vi "Begin.vi"(8 "error in":errorcluster) -> (0 "error out":errorcluster)   [LabVIEW 2020]
doc: "Called before other user functions, this VI is expected to open initial I/O refnums, load in file data, and do all program initialization. Notice that the <B>error out</B> terminal is simply used for data flow. Wiring it to other structures or subVIs ensures that this VI runs first."
uses:
  <vilib>/Rock Robotics/WPI/DriverStation/WPI_DriverStationRobotMode2.ctl
  <vilib>/Rock Robotics/WPI/Joystick/WPI_JoystickDeviceEnum.ctl
  <vilib>/Rock Robotics/WPI/ThirdParty/REV Robotics/REVLib/Typedef/Spark MAX Motor Type.ctl
  <vilib>/Rock Robotics/WPI/SafetyOutput/WPI_SafetyOutputConfigMenu.ctl
  <vilib>/Rock Robotics/SystemInterfaces/DIO/FPGA_DIOChannel.ctl
  <vilib>/Rock Robotics/WPI/Encoder/WPI_EncoderType.ctl
  <vilib>/Rock Robotics/SystemInterfaces/spilib/spi_bus.ctl
  <vilib>/Rock Robotics/WPI/Solenoid/WPI_SolenoidChannel.ctl
  <vilib>/Rock Robotics/WPI/ThirdParty/REV Robotics/REVLib/Typedef/Spark MAX Idle Mode.ctl
  <vilib>/Rock Robotics/WPI/ThirdParty/Phoenix-LabVIEW/Motor Controller/Controls/CTRE_Phoenix_MotorControl_ControlMode.ctl
  <vilib>/Rock Robotics/WPI/DriverStation/WPI_DriverStationAllianceInfo.ctl
  <vilib>/Rock Robotics/SystemInterfaces/i2clib/i2c_bus.ctl
  Robot Global Data.vi
  <vilib>/Rock Robotics/Network Tables/NT Write String Array.vi
  <vilib>/Rock Robotics/WPI/Counter/WPI_CounterDigitalInputToDigitalSource.vi
  <vilib>/Rock Robotics/WPI/Gyro/WPI_GyroXRS450_SPI_Open.vi
  <vilib>/Rock Robotics/WPI/Solenoid/WPI_SolenoidOpenDouble.vi
  <vilib>/Rock Robotics/WPI/Switch/WPI_SwitchOpenLimit.vi
  Global Variable/StateMachineOperation.vi
  <vilib>/Rock Robotics/WPI/Utilities/WPI_GetSetVariantRefNum.vi
panel:
  in  "Nothing":cluster{"R":dbl, "G":dbl, "B":dbl}={"R"=0.197, "G"=0.561, "B"=0.24}
  in  "Red Calibration":cluster{"R":dbl, "G":dbl, "B":dbl}={"R"=0.561, "G"=0.323, "B"=0.114}
  in  "Blue Calibration":cluster{"R":dbl, "G":dbl, "B":dbl}={"R"=0.143, "G"=0.427, "B"=0.429}
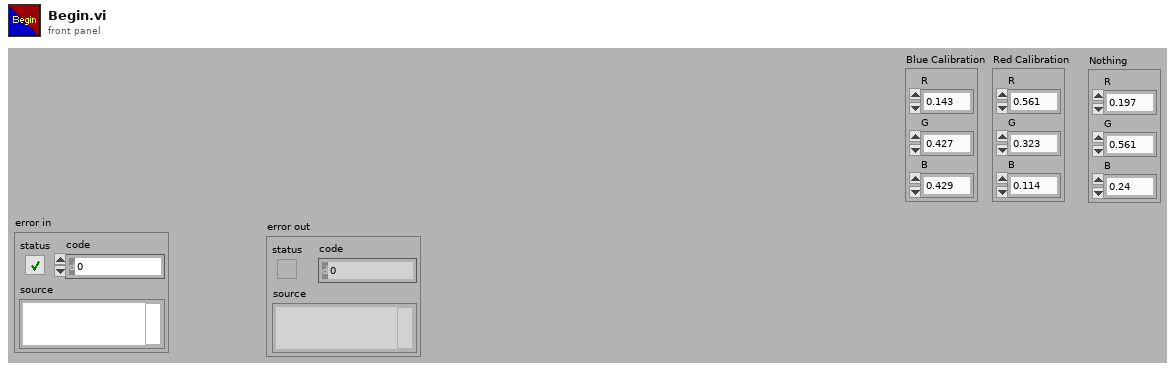
[diagram p1: front panel]
types:
  T1 = typedef "FPGA_DIOChannel.ctl" = enum8{"DIO 0", "DIO 1", "DIO 2", "DIO 3", "DIO 4", "DIO 5", "DIO 6", "DIO 7", "DIO 8", "DIO 9", "DIO MXP 0", "DIO MXP 1", "DIO MXP 2", "DIO MXP 3", "DIO MXP 4", "DIO MXP 5", "DIO MXP 6", "DIO MXP 7", "DIO MXP 8", "DIO MXP 9", "DIO MXP 10", "DIO MXP 11", "DIO MXP 12", "DIO MXP 13", "DIO MXP 14", "DIO MXP 15", "SPI Port CS1", "SPI Port CS2", "SPI Port CS3", "SPI Port MISO", "SPI Port MOSI", "Invalid"}
  T2 = typedef "i2c_bus.ctl" = enum16{"I2C On-Board", "I2C MXP", "Invalid"}
  T3 = typedef "WPI_DriverStationAllianceInfo.ctl" = enum16{"Red", "Blue", "Invalid"}
  T4 = typedef "WPI_EncoderType.ctl" = enum16{"1x", "2x", "4x"}
  T5 = typedef "Spark MAX Motor Type.ctl" = enum16{"Brushed", "Brushless"}
  T6 = typedef "Spark MAX Idle Mode.ctl" = enum16{"Coast", "Brake"}
  T7 = typedef "CTRE_Phoenix_MotorControl_ControlMode.ctl" = u16
  T8 = typedef "WPI_SolenoidChannel.ctl" = enum8{"Solenoid 0", "Solenoid 1", "Solenoid 2", "Solenoid 3", "Solenoid 4", "Solenoid 5", "Solenoid 6", "Solenoid 7", "Solenoid 8", "Solenoid 9", "Solenoid 10", "Solenoid 11", "Solenoid 12", "Solenoid 13", "Solenoid 14", "Solenoid 15", "Invalid"}
  T9 = typedef "spi_bus.ctl" = enum16{"SPI On-Board, CS0", "SPI On-Board, CS1", "SPI On-Board, CS2", "SPI On-Board, CS3", "SPI MXP", "Invalid"}
  T10 = typedef "WPI_SafetyOutputConfigMenu.ctl" = enum16{"Enable", "Disable"}
  T11 = typedef "WPI_JoystickDeviceEnum.ctl" = enum16{"USB 0", "USB 1", "USB 2", "USB 3", "USB 4", "USB 5"}
  T12 = typedef "WPI_DriverStationRobotMode2.ctl" = enum16{"Autonomous Disabled", "Autonomous Enabled", "Teleop Disabled", "Teleop Enabled", "Disconnected", "Finish", "Test Disabled", "Test Enabled", "Emergency Stopped"}
  T13 = typedef "WPI_MotorControlDeviceRef.ctl" = cluster{"DeviceStatus":errorcluster, "Type":T14, "PWM":cluster{"PWM Channel":T15, "DeadBand":T16}, "CAN":cluster{"Device Number":u8, "SetOutput VI Ref":variant, "GetOutput VI Ref":variant, "Enable VI Ref":variant, "Disable VI Ref":variant, "Data":variant}, "Invert":bool, "DIO PWM":cluster{"PWM \"Enable\" Channel":T15, "DIOChannel":T1, "PWM Rate":dbl}}
  T14 = typedef "WPI_MotorControlType.ctl" = enum16{"PWM", "CAN", "DIO PWM"}
  T15 = typedef "FPGA_DIOPWMChannel.ctl" = enum8{"PWM 0", "PWM 1", "PWM 2", "PWM 3", "PWM 4", "PWM 5", "PWM 6", "PWM 7", "PWM 8", "PWM 9", "PWM MXP 0", "PWM MXP 1", "PWM MXP 2", "PWM MXP 3", "PWM MXP 4", "PWM MXP 5", "PWM MXP 6", "PWM MXP 7", "PWM MXP 8", "PWM MXP 9", "Invalid"}
  T16 = typedef "WPI_PWMDeadband.ctl" = cluster{"Name":string, "maxPositivePwm":i32, "minPositivePwm":i32, "centerPwm":i32, "maxNegativePwm":i32, "minNegativePwm":i32, "angularRange":u16}
  T17 = typedef "WPI_JoystickDevRef.ctl" = cluster{"Device":T11}
  T18 = typedef "WPI_DigitalInputDevRef.ctl" = cluster{"DevStatus":errorcluster, "DIO Channel":T1}
  T19 = typedef "FPGA_CounterEncoderSourceConvertionLVSourceType.ctl" = cluster{"DevStatus":errorcluster, "AnalogTriggerMode?":bool, "DigitalMode":cluster{"DIO Channel":T20}, "AnalogTriggerMode":cluster{"AnalogTriggerIndex":T21, "OutputType":T22}}
  T20 = typedef "FPGA_DIODigitalSourceChannel.ctl" = enum8{"DIO 0", "DIO 1", "DIO 2", "DIO 3", "DIO 4", "DIO 5", "DIO 6", "DIO 7", "DIO 8", "DIO 9", "DIO MXP 0", "DIO MXP 1", "DIO MXP 2", "DIO MXP 3", "DIO MXP 4", "DIO MXP 5", "DIO MXP 6", "DIO MXP 7", "DIO MXP 8", "DIO MXP 9", "DIO MXP 10", "DIO MXP 11", "DIO MXP 12", "DIO MXP 13", "DIO MXP 14", "DIO MXP 15", "SPI Port CS1", "SPI Port CS2", "SPI Port CS3", "SPI Port MISO", "SPI Port MOSI", "Disabled"}
  T21 = typedef "FPGA_AnalogTriggerIndex.ctl" = enum8{"Trig 0", "Trig 1", "Trig 2", "Trig 3", "Trig 4", "Trig 5", "Trig 6", "Trig 7", "Invalid"}
  T22 = typedef "FPGA_AnalogTriggerOutType.ctl" = enum16{"InWindow", "TriggerState", "Rising", "Falling"}
  T23 = typedef "WPI_EncoderDevRef.ctl" = cluster{"DevStatus":errorcluster, "EncoderIndex":T24, "CounterIndex":T25, "DistancePerCount":dbl, "Decoding Type":T4}
  T24 = typedef "FPGA_EncoderIdx.ctl" = enum8{"Enc 0", "Enc 1", "Enc 2", "Enc 3", "Enc 4", "Enc 5", "Enc 6", "Enc 7", "Invalid"}
  T25 = typedef "FPGA_CounterCtrSystemIndex.ctl" = enum8{"Ctr 0", "Ctr 1", "Ctr 2", "Ctr 3", "Ctr 4", "Ctr 5", "Ctr 6", "Ctr 7", "Invalid"}
  T26 = typedef "WPI_GyroDevRef.ctl" = cluster{"DevStatus":errorcluster, "Analog Channel":T27, "Gain (VoltsPerDegree/Second)":dbl, "Gyro Type":enum16{"Analog", "XRS450"}, "Handle":i32, "SPI Bus":T9, "Device Found":bool, "Sample Rate":dbl, "Calibrate On Open":bool, "Offset":dbl}
  T27 = typedef "FPGA_AIChannel.ctl" = enum8{"AI 0", "AI 1", "AI 2", "AI 3", "AI MXP 0", "AI MXP 1", "AI MXP 2", "AI MXP 3", "Invalid"}
  T28 = typedef "WPI_CompressorDevRef.ctl" = cluster{"DevStatus":errorcluster, "Pneumatics Control Module":u8}
  T29 = typedef "Color Sensor V3 DevRef.ctl" = cluster{"I2CDevRef":T30}
  T30 = typedef "WPI_I2CDevRef.ctl" = cluster{"DevStatus":errorcluster, "Device Address":u8, "Handle":i32, "I2C Bus":T2}
  T31 = typedef "WPI_SwitchDevRef.ctl" = cluster{"DevStatus":errorcluster, "DIO Channel":T1, "CntIndex":T25, "Normally Closed":bool}
  T32 = typedef "WPI_SolenoidDevRef.ctl" = cluster{"DevStatus":errorcluster, "Pneumatics Control Module":u8, "Forward Solenoid Channel":T8, "Reverse Solenoid Channel":T8}
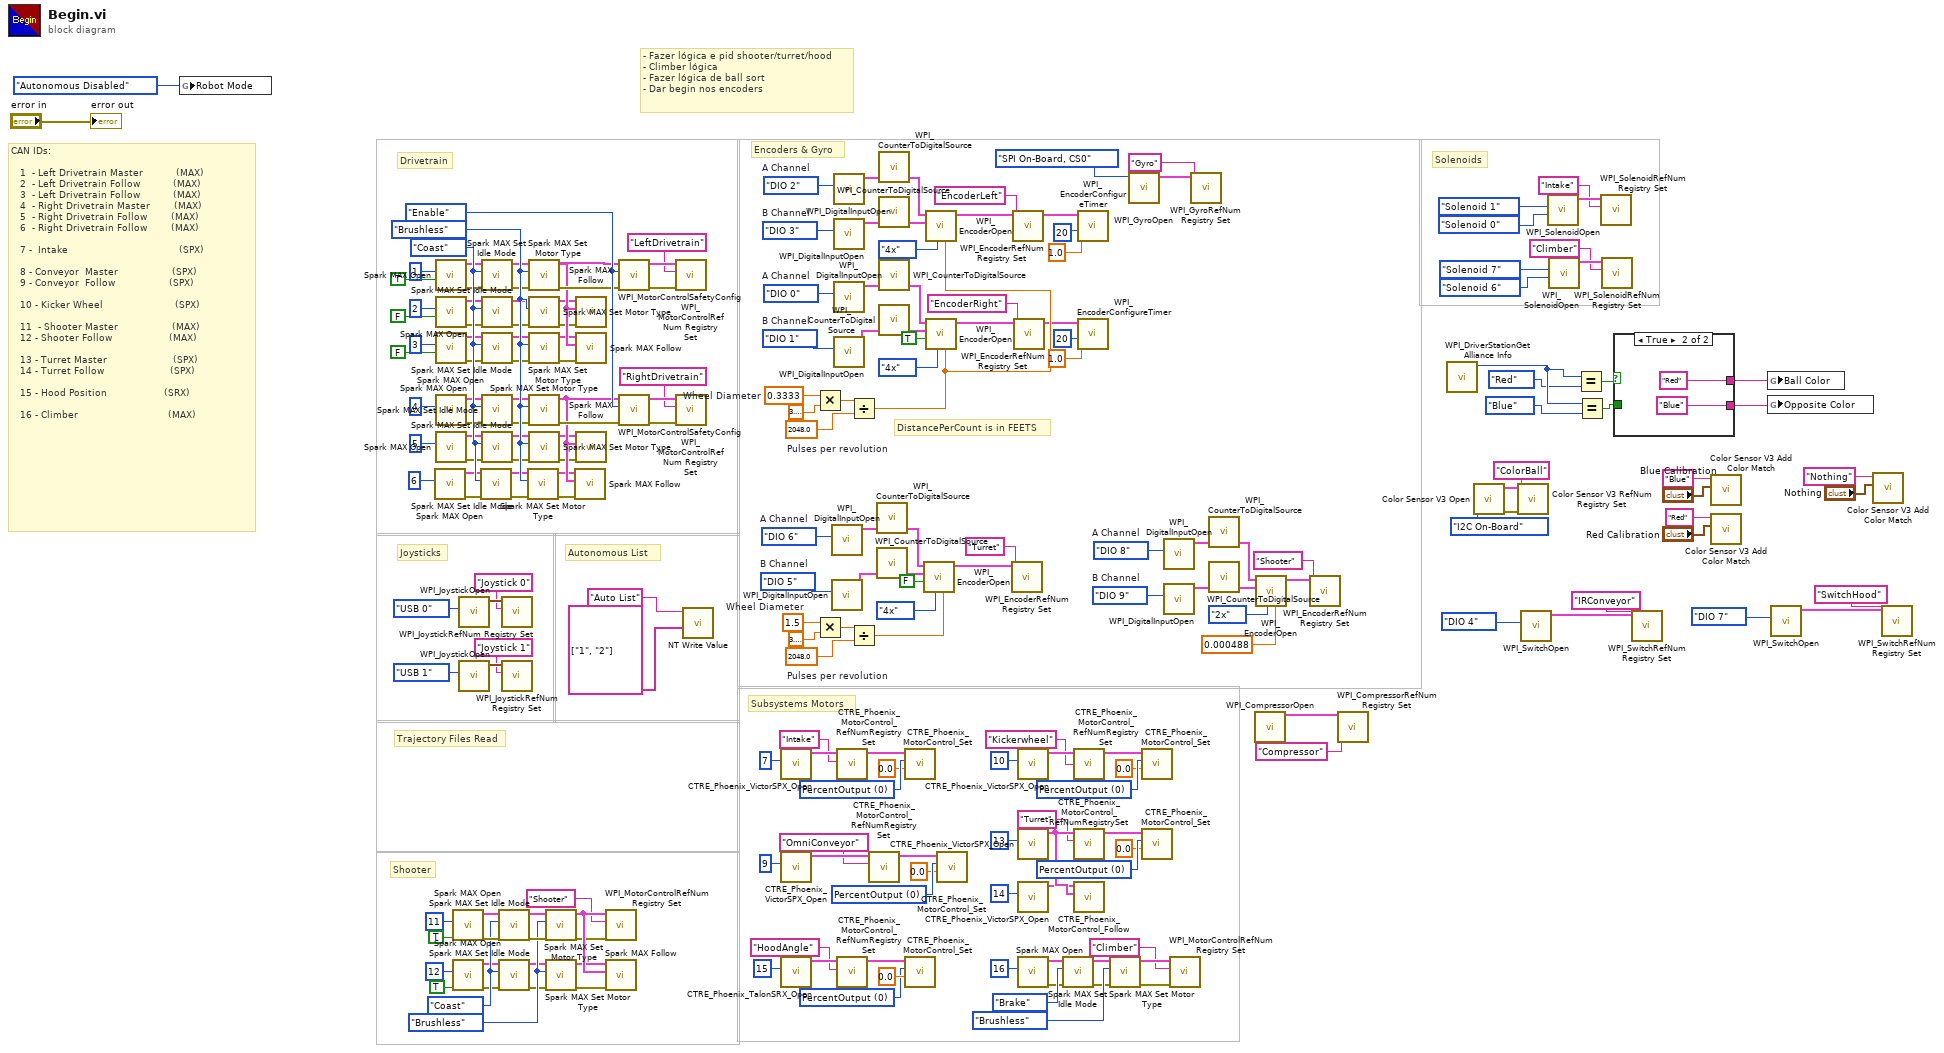
[diagram p0: block diagram]
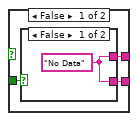
[diagram p2: hidden frame]
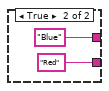
[diagram p3: hidden frame]
diagram:
  w6 = dbl[unit] 2048.0  # Pulses per revolution
  w9 = dbl[unit] 1.5  # Wheel Diameter
  w58 = FPGA_DIOChannel."DIO 9"  # B Channel
  w57 = FPGA_DIOChannel."DIO 8"  # A Channel
  w66 = FPGA_DIOChannel."DIO 5"  # B Channel
  w65 = FPGA_DIOChannel."DIO 6"  # A Channel
  w79 = T7 0 items=["PercentOutput"=0, "Position"=1, "Velocity"=2, "Current"=3, "Follower"=5, "MotionProfile"=6, "MotionMagic"=7, "MotionProfileArc"=10, "Disabled"=15] ("Control Mode")
  w86 = T7 0 items=["PercentOutput"=0, "Position"=1, "Velocity"=2, "Current"=3, "Follower"=5, "MotionProfile"=6, "MotionMagic"=7, "MotionProfileArc"=10, "Disabled"=15] ("Control Mode")
  w92 = Spark_MAX_Motor_Type."Brushless" ("Motor Type")
  w93 = Spark_MAX_Idle_Mode."Coast" ("Idle Mode")
  w102 = T7 0 items=["PercentOutput"=0, "Position"=1, "Velocity"=2, "Current"=3, "Follower"=5, "MotionProfile"=6, "MotionMagic"=7, "MotionProfileArc"=10, "Disabled"=15] ("Control Mode")
  w116 = T7 0 items=["PercentOutput"=0, "Position"=1, "Velocity"=2, "Current"=3, "Follower"=5, "MotionProfile"=6, "MotionMagic"=7, "MotionProfileArc"=10, "Disabled"=15] ("Control Mode")
  w122 = T7 0 items=["PercentOutput"=0, "Position"=1, "Velocity"=2, "Current"=3, "Follower"=5, "MotionProfile"=6, "MotionMagic"=7, "MotionProfileArc"=10, "Disabled"=15] ("Control Mode")
  w180 = dbl[unit] 2048.0  # Pulses per revolution
  w183 = dbl[unit] 0.3333  # Wheel Diameter
  w190 = FPGA_DIOChannel."DIO 1"  # B Channel
  w189 = FPGA_DIOChannel."DIO 0"  # A Channel
  w199 = FPGA_DIOChannel."DIO 3"  # B Channel
  w198 = FPGA_DIOChannel."DIO 2"  # A Channel
  w206 = WPI_SafetyOutputConfigMenu."Enable" ("mode")
  w173 = Spark_MAX_Motor_Type."Brushless" ("Motor Type")
  w174 = Spark_MAX_Idle_Mode."Coast" ("Idle Mode")
  # "Solenoids"
  # "Subsystems Motors"
  # "Shooter"
  # "- Fazer lógica e pid shooter/turret/hood\n- Climber lógica\n- Fazer lógica de ball sort \n- Dar begin nos encoders"
  # "Trajectory Files Read"
  # "DistancePerCount is in FEETS"
  # "Encoders & Gyro"
  # "Drivetrain"
  # "Autonomous List"
  # "Joysticks"
  # "CAN IDs:\n\n   1  - Left Drivetrain Master           (MAX)\n   2  - Left Drivetrain Follow           (MAX)\n   3  - Left Drivetrain Follow           (MAX)\n   4  - Right Drivetrain Master        (MAX)\n   5  - Right Drivetrain Follow        (MAX)\n   6  - Right Drivetrain Follow        (MAX)\n\n   7 -  Intake                                     (SPX)\n\n   8 - Conveyor  Master                  (SPX)\n   9 - Conveyor  Follow                  (SPX)\n\n   10 - Kicker Wheel                        (SPX)\n\n   11  - Shooter Master                  (MAX)\n   12 - Shooter Follow                   (MAX)\n\n   13 - Turret Master                      (SPX)\n   14 - Turret Follow                      (SPX)\n\n   15 - Hood Position                   (SRX)\n\n   16 - Climber                              (MAX)"
  n1 = global write "Robot Global Data.vi" "Robot Mode"(WPI_DriverStationRobotMode2."Autonomous Disabled" ("Robot Mode")) -> ()
  n2 = call <vilib>:"Spark MAX Open.vi"("Device Number"=u8 6) -> ("error out"=w155:errorcluster, "MotorControlDeviceRef"=w152:T13)  [unwired: 9 in]
  n3 = call <vilib>:"Spark MAX Open.vi"("Invert"=TRUE, "Device Number"=u8 1) -> ("error out"=w145:errorcluster, "MotorControlDeviceRef"=w147:T13)  [unwired: 8 in]
  n4 = call <vilib>:"Spark MAX Open.vi"("Invert"=FALSE, "Device Number"=u8 2) -> ("error out"=w140:errorcluster, "MotorControlDeviceRef"=w128:T13)  [unwired: 8 in]
  n5 = call <vilib>:"Spark MAX Open.vi"("Invert"=FALSE, "Device Number"=u8 3) -> ("error out"=w136:errorcluster, "MotorControlDeviceRef"=w133:T13)  [unwired: 8 in]
  n6 = call <vilib>:"Spark MAX Open.vi"("Device Number"=u8 4) -> ("error out"=w166:errorcluster, "MotorControlDeviceRef"=w163:T13)  [unwired: 9 in]
  n7 = call <vilib>:"Spark MAX Open.vi"("Device Number"=u8 5) -> ("error out"=w160:errorcluster, "MotorControlDeviceRef"=w150:T13)  [unwired: 9 in]
  n8 = call <vilib>:"Spark MAX Open.vi"("Invert"=TRUE, "Device Number"=u8 11) -> ("error out"=w96:errorcluster, "MotorControlDeviceRef"=w98:T13)  [unwired: 8 in]
  n9 = call <vilib>:"Spark MAX Open.vi"("Invert"=TRUE, "Device Number"=u8 12) -> ("error out"=w13:errorcluster, "MotorControlDeviceRef"=w17:T13)  [unwired: 8 in]
  n10 = call <vilib>:"WPI_JoystickOpen.vi"("JoystickDevice"=WPI_JoystickDeviceEnum."USB 0") -> ("JoystickDevRef"=w211:T17)  [unwired: 10 in]
  n11 = call <vilib>:"WPI_JoystickOpen.vi"("JoystickDevice"=WPI_JoystickDeviceEnum."USB 1") -> ("JoystickDevRef"=w208:T17)  [unwired: 10 in]
  n12 = call <vilib>:"Spark MAX Set Idle Mode.vi"("error in (no error)"=w155, "Idle Mode"=w174, "MotorControlDeviceRef in"=w152) -> ("error out"=w154:errorcluster, "MotorControlDeviceRef out"=w151:T13)  [unwired: 7 in]
  n13 = call <vilib>:"Spark MAX Set Idle Mode.vi"("error in (no error)"=w145, "Idle Mode"=w174, "MotorControlDeviceRef in"=w147) -> ("error out"=w144:errorcluster, "MotorControlDeviceRef out"=w146:T13)  [unwired: 7 in]
  n14 = call <vilib>:"Spark MAX Set Idle Mode.vi"("error in (no error)"=w140, "Idle Mode"=w174, "MotorControlDeviceRef in"=w128) -> ("error out"=w139:errorcluster, "MotorControlDeviceRef out"=w127:T13)  [unwired: 7 in]
  n15 = call <vilib>:"Spark MAX Set Idle Mode.vi"("error in (no error)"=w136, "Idle Mode"=w174, "MotorControlDeviceRef in"=w133) -> ("error out"=w135:errorcluster, "MotorControlDeviceRef out"=w132:T13)  [unwired: 7 in]
  n16 = call <vilib>:"Spark MAX Set Idle Mode.vi"("error in (no error)"=w166, "Idle Mode"=w174, "MotorControlDeviceRef in"=w163) -> ("error out"=w165:errorcluster, "MotorControlDeviceRef out"=w164:T13)  [unwired: 7 in]
  n17 = call <vilib>:"Spark MAX Set Idle Mode.vi"("error in (no error)"=w160, "Idle Mode"=w174, "MotorControlDeviceRef in"=w150) -> ("error out"=w159:errorcluster, "MotorControlDeviceRef out"=w149:T13)  [unwired: 7 in]
  n18 = call <vilib>:"Spark MAX Set Idle Mode.vi"("error in (no error)"=w96, "Idle Mode"=w93, "MotorControlDeviceRef in"=w98) -> ("error out"=w100:errorcluster, "MotorControlDeviceRef out"=w95:T13)  [unwired: 7 in]
  n19 = call <vilib>:"Spark MAX Set Idle Mode.vi"("error in (no error)"=w13, "Idle Mode"=w93, "MotorControlDeviceRef in"=w17) -> ("error out"=w19:errorcluster, "MotorControlDeviceRef out"=w14:T13)  [unwired: 7 in]
  n20 = call <vilib>:"WPI_JoystickRefNum Registry Set.vi"("refnum name"="Joystick 0", "JoystickDevRef"=w211) -> ()  [unwired: 8 in, 2 out]
  n21 = call <vilib>:"WPI_JoystickRefNum Registry Set.vi"("refnum name"="Joystick 1", "JoystickDevRef"=w208) -> ()  [unwired: 8 in, 2 out]
  n22 = call <vilib>:"Spark MAX Set Motor Type.vi"("error in (no error)"=w154, "Motor Type"=w173, "MotorControlDevRef"=w151) -> ("error out"=w153:errorcluster, "MotorControlDeviceRef"=w156:T13)  [unwired: 7 in]
  n23 = call <vilib>:"Spark MAX Set Motor Type.vi"("error in (no error)"=w144, "Motor Type"=w173, "MotorControlDevRef"=w146) -> ("error out"=w203:errorcluster, "MotorControlDeviceRef"=w175:T13)  [unwired: 7 in]
  n24 = call <vilib>:"Spark MAX Set Motor Type.vi"("error in (no error)"=w139, "Motor Type"=w173, "MotorControlDevRef"=w127) -> ("error out"=w138:errorcluster, "MotorControlDeviceRef"=w141:T13)  [unwired: 7 in]
  n25 = call <vilib>:"Spark MAX Set Motor Type.vi"("error in (no error)"=w135, "Motor Type"=w173, "MotorControlDevRef"=w132) -> ("error out"=w134:errorcluster, "MotorControlDeviceRef"=w131:T13)  [unwired: 7 in]
  n26 = call <vilib>:"Spark MAX Set Motor Type.vi"("error in (no error)"=w165, "Motor Type"=w173, "MotorControlDevRef"=w164) -> ("error out"=w170:errorcluster, "MotorControlDeviceRef"=w168:T13)  [unwired: 7 in]
  n27 = call <vilib>:"Spark MAX Set Motor Type.vi"("error in (no error)"=w159, "Motor Type"=w173, "MotorControlDevRef"=w149) -> ("error out"=w158:errorcluster, "MotorControlDeviceRef"=w161:T13)  [unwired: 7 in]
  n28 = call <vilib>:"Spark MAX Set Motor Type.vi"("error in (no error)"=w100, "Motor Type"=w92, "MotorControlDevRef"=w95) -> ("error out"=w94:errorcluster, "MotorControlDeviceRef"=w97:T13)  [unwired: 7 in]
  n29 = call <vilib>:"Spark MAX Set Motor Type.vi"("error in (no error)"=w19, "Motor Type"=w92, "MotorControlDevRef"=w14) -> ("error out"=w15:errorcluster, "MotorControlDeviceRef"=w16:T13)  [unwired: 7 in]
  n30 = call <vilib>:"Spark MAX Follow.vi"("error in (no error)"=w153, "Master Controller"=w168, "MotorControlDeviceRef"=w156) -> ()  [unwired: 7 in, 2 out]
  n31 = call <vilib>:"Spark MAX Follow.vi"("error in (no error)"=w138, "Master Controller"=w175, "MotorControlDeviceRef"=w141) -> ()  [unwired: 7 in, 2 out]
  n32 = call <vilib>:"Spark MAX Follow.vi"("error in (no error)"=w134, "Master Controller"=w175, "MotorControlDeviceRef"=w131) -> ()  [unwired: 7 in, 2 out]
  n33 = call <vilib>:"Spark MAX Follow.vi"("error in (no error)"=w158, "Master Controller"=w168, "MotorControlDeviceRef"=w161) -> ()  [unwired: 7 in, 2 out]
  n34 = call <vilib>:"WPI_MotorControlRefNum Registry Set.vi"("error in (no error)"=w94, "refnum name"="Shooter", "MotorControlDevRef"=w97) -> ()  [unwired: 7 in, 2 out]
  n35 = call <vilib>:"Spark MAX Follow.vi"("error in (no error)"=w15, "Master Controller"=w97, "MotorControlDeviceRef"=w16) -> ()  [unwired: 7 in, 2 out]
  n36 = call <vilib>:"WPI_MotorControlSafetyConfig.vi"("error in (no error)"=w203, "mode"=w206, "MotorControlDevRef"=w175) -> ("error out"=w202:errorcluster, "MotorControlDevRef"=w205:T13)  [unwired: 7 in]
  n37 = call <vilib>:"WPI_MotorControlSafetyConfig.vi"("error in (no error)"=w170, "mode"=w206, "MotorControlDevRef"=w168) -> ("error out"=w169:errorcluster, "MotorControlDevRef"=w172:T13)  [unwired: 7 in]
  n38 = call <vilib>:"WPI_MotorControlRefNum Registry Set.vi"("error in (no error)"=w202, "refnum name"="LeftDrivetrain", "MotorControlDevRef"=w205) -> ()  [unwired: 7 in, 2 out]
  n39 = call <vilib>:"WPI_MotorControlRefNum Registry Set.vi"("error in (no error)"=w169, "refnum name"="RightDrivetrain", "MotorControlDevRef"=w172) -> ()  [unwired: 7 in, 2 out]
  n40 = call-poly <vilib>:"NT Write Value.vi"("String Array"=string[] ["1", "2"], "Name"="Auto List") -> ()  [unwired: 9 in, 1 out]
  n41 = call <vilib>:"CTRE_Phoenix_VictorSPX_Open.vi"("Device Number"=u8 7) -> ("PhoenixMotorControlDevRef"=w120:T13)  [unwired: 9 in, 1 out]
  n42 = call <vilib>:"CTRE_Phoenix_VictorSPX_Open.vi"("Device Number"=u8 9) -> ("PhoenixMotorControlDevRef"=w126:T13)  [unwired: 9 in, 1 out]
  n43 = call <vilib>:"CTRE_Phoenix_TalonSRX_Open.vi"("Device Number"=u8 15) -> ("PhoenixMotorControlDevRef"=w84:T13)  [unwired: 9 in, 1 out]
  n44 = Multiply(x=w183, y=3.141592653589793) -> (x*y=w181:dbl[unit])
  n45 = Multiply(x=w9, y=3.141592653589793) -> (x*y=w7:dbl[unit])
  n46 = call <vilib>:"WPI_DigitalInputOpen.vi"("DIO Channel"=w65) -> ("DigitalInputDevRef"=w63:T18)  [unwired: 1 in, 9 out]
  n47 = call <vilib>:"WPI_DigitalInputOpen.vi"("DIO Channel"=w66) -> ("DigitalInputDevRef"=w64:T18)  [unwired: 1 in, 9 out]
  n48 = call <vilib>:"WPI_DigitalInputOpen.vi"("DIO Channel"=w198) -> ("DigitalInputDevRef"=w196:T18)  [unwired: 1 in, 9 out]
  n49 = call <vilib>:"WPI_DigitalInputOpen.vi"("DIO Channel"=w199) -> ("DigitalInputDevRef"=w197:T18)  [unwired: 1 in, 9 out]
  n50 = call <vilib>:"WPI_DigitalInputOpen.vi"("DIO Channel"=w189) -> ("DigitalInputDevRef"=w187:T18)  [unwired: 1 in, 9 out]
  n51 = call <vilib>:"WPI_DigitalInputOpen.vi"("DIO Channel"=w190) -> ("DigitalInputDevRef"=w188:T18)  [unwired: 1 in, 9 out]
  n52 = call <vilib>:"CTRE_Phoenix_MotorControl_RefNumRegistrySet.vi"("refnum name"="Intake", "PhoenixMotorControlDevRef"=w120) -> ("PhoenixMotorControlDevRef"=w117:T13)  [unwired: 8 in, 1 out]
  n53 = call <vilib>:"CTRE_Phoenix_MotorControl_RefNumRegistrySet.vi"("refnum name"="HoodAngle", "PhoenixMotorControlDevRef"=w84) -> ("PhoenixMotorControlDevRef"=w81:T13)  [unwired: 8 in, 1 out]
  n54 = Divide(x=w181, y=w180) -> (x/y=w179:dbl)
  n55 = Divide(x=w7, y=w6) -> (x/y=w5:dbl)
  n56 = call <vilib>:"CTRE_Phoenix_MotorControl_RefNumRegistrySet.vi"("refnum name"="OmniConveyor", "PhoenixMotorControlDevRef"=w126) -> ("PhoenixMotorControlDevRef"=w123:T13)  [unwired: 8 in, 1 out]
  n57 = call-poly <vilib>:"WPI_CounterToDigitalSource.vi"("DigitalInputDevRef"=w63) -> ("Digital Source"=w67:T19)  [unwired: 6 out]
  n58 = call-poly <vilib>:"WPI_CounterToDigitalSource.vi"("DigitalInputDevRef"=w64) -> ("Digital Source"=w68:T19)  [unwired: 6 out]
  n59 = call-poly <vilib>:"WPI_CounterToDigitalSource.vi"("DigitalInputDevRef"=w196) -> ("Digital Source"=w200:T19)  [unwired: 6 out]
  n60 = call-poly <vilib>:"WPI_CounterToDigitalSource.vi"("DigitalInputDevRef"=w197) -> ("Digital Source"=w201:T19)  [unwired: 6 out]
  n61 = call-poly <vilib>:"WPI_CounterToDigitalSource.vi"("DigitalInputDevRef"=w187) -> ("Digital Source"=w191:T19)  [unwired: 6 out]
  n62 = call-poly <vilib>:"WPI_CounterToDigitalSource.vi"("DigitalInputDevRef"=w188) -> ("Digital Source"=w192:T19)  [unwired: 6 out]
  n63 = call <vilib>:"CTRE_Phoenix_MotorControl_Set.vi"("Output"=0.0, "Control Mode"=w116, "PhoenixMotorControlDevRef"=w117) -> ()  [unwired: 7 in, 2 out]
  n64 = call <vilib>:"CTRE_Phoenix_MotorControl_Set.vi"("Output"=0.0, "Control Mode"=w79, "PhoenixMotorControlDevRef"=w81) -> ()  [unwired: 7 in, 2 out]
  n65 = call <vilib>:"WPI_EncoderOpen.vi"("DistancePerCount"=w5, "Decoding Type"=WPI_EncoderType."4x", "Invert Direction (False)"=FALSE, "BSource"=w68, "ASource"=w67) -> ("EncoderDevRef"=w62:T23)  [unwired: 5 in, 1 out]
  n66 = call <vilib>:"WPI_EncoderOpen.vi"("DistancePerCount"=w179, "Decoding Type"=WPI_EncoderType."4x", "BSource"=w201, "ASource"=w200) -> ("EncoderDevRef"=w195:T23)  [unwired: 6 in, 1 out]
  n67 = call <vilib>:"WPI_EncoderOpen.vi"("DistancePerCount"=w179, "Decoding Type"=WPI_EncoderType."4x", "Invert Direction (False)"=TRUE, "BSource"=w192, "ASource"=w191) -> ("EncoderDevRef"=w186:T23)  [unwired: 5 in, 1 out]
  n68 = call <vilib>:"CTRE_Phoenix_MotorControl_Set.vi"("Output"=0.0, "Control Mode"=w122, "PhoenixMotorControlDevRef"=w123) -> ()  [unwired: 7 in, 2 out]
  n69 = call <vilib>:"WPI_EncoderRefNum Registry Set.vi"("refnum name"="Turret", "EncoderDevRef"=w62) -> ()  [unwired: 8 in, 2 out]
  n70 = call <vilib>:"WPI_EncoderRefNum Registry Set.vi"("refnum name"="EncoderLeft", "EncoderDevRef"=w195) -> ("EncoderDevRef"=w47:T23)  [unwired: 8 in, 1 out]
  n71 = call <vilib>:"WPI_EncoderRefNum Registry Set.vi"("refnum name"="EncoderRight", "EncoderDevRef"=w186) -> ("EncoderDevRef"=w46:T23)  [unwired: 8 in, 1 out]
  n72 = call <vilib>:"CTRE_Phoenix_VictorSPX_Open.vi"("Device Number"=u8 10) -> ("PhoenixMotorControlDevRef"=w106:T13)  [unwired: 9 in, 1 out]
  n73 = call <vilib>:"CTRE_Phoenix_VictorSPX_Open.vi"("Device Number"=u8 13) -> ("PhoenixMotorControlDevRef"=w90:T13)  [unwired: 9 in, 1 out]
  n74 = call <vilib>:"CTRE_Phoenix_VictorSPX_Open.vi"("Device Number"=u8 14) -> ("PhoenixMotorControlDevRef"=w24:T13)  [unwired: 9 in, 1 out]
  n75 = call <vilib>:"Spark MAX Open.vi"("Device Number"=u8 16) -> ("error out"=w71:errorcluster, "MotorControlDeviceRef"=w77:T13)  [unwired: 9 in]
  n76 = call <vilib>:"Spark MAX Set Idle Mode.vi"("error in (no error)"=w71, "Idle Mode"=Spark_MAX_Idle_Mode."Brake", "MotorControlDeviceRef in"=w77) -> ("error out"=w70:errorcluster, "MotorControlDeviceRef out"=w75:T13)  [unwired: 7 in]
  n77 = call <vilib>:"CTRE_Phoenix_MotorControl_RefNumRegistrySet.vi"("refnum name"="Kickerwheel", "PhoenixMotorControlDevRef"=w106) -> ("PhoenixMotorControlDevRef"=w103:T13)  [unwired: 8 in, 1 out]
  n78 = call <vilib>:"CTRE_Phoenix_MotorControl_RefNumRegistrySet.vi"("refnum name"="Turret", "PhoenixMotorControlDevRef"=w90) -> ("PhoenixMotorControlDevRef"=w87:T13)  [unwired: 8 in, 1 out]
  n79 = call <vilib>:"CTRE_Phoenix_MotorControl_Follow.vi"("Master Controller to Follow"=w90, "PhoenixMotorControlDevRef"=w24) -> ()  [unwired: 8 in, 2 out]
  n80 = call <vilib>:"WPI_EncoderConfigureTimer.vi"("Number Samples to Average"=u8 20, "Minimum Rate"=1.0, "EncoderDevRef"=w47) -> ()  [unwired: 7 in, 2 out]
  n81 = call <vilib>:"WPI_EncoderConfigureTimer.vi"("Number Samples to Average"=u8 20, "Minimum Rate"=1.0, "EncoderDevRef"=w46) -> ()  [unwired: 7 in, 2 out]
  n82 = call <vilib>:"Spark MAX Set Motor Type.vi"("error in (no error)"=w70, "Motor Type"=Spark_MAX_Motor_Type."Brushless", "MotorControlDevRef"=w75) -> ("error out"=w69:errorcluster, "MotorControlDeviceRef"=w76:T13)  [unwired: 7 in]
  n83 = call-poly <vilib>:"WPI_GyroOpen.vi"("SPI Bus"=spi_bus."SPI On-Board, CS0") -> ("GyroDevRef"=w178:T26)  [unwired: 8 in, 2 out]
  n84 = call <vilib>:"CTRE_Phoenix_MotorControl_Set.vi"("Output"=0.0, "Control Mode"=w102, "PhoenixMotorControlDevRef"=w103) -> ()  [unwired: 7 in, 2 out]
  n85 = call <vilib>:"CTRE_Phoenix_MotorControl_Set.vi"("Output"=0.0, "Control Mode"=w86, "PhoenixMotorControlDevRef"=w87) -> ()  [unwired: 7 in, 2 out]
  n86 = call <vilib>:"WPI_DigitalInputOpen.vi"("DIO Channel"=w57) -> ("DigitalInputDevRef"=w55:T18)  [unwired: 1 in, 9 out]
  n87 = call <vilib>:"WPI_DigitalInputOpen.vi"("DIO Channel"=w58) -> ("DigitalInputDevRef"=w56:T18)  [unwired: 1 in, 9 out]
  n88 = call <vilib>:"WPI_MotorControlRefNum Registry Set.vi"("error in (no error)"=w69, "refnum name"="Climber", "MotorControlDevRef"=w76) -> ()  [unwired: 7 in, 2 out]
  n89 = call <vilib>:"WPI_GyroRefNum Registry Set.vi"("refnum name"="Gyro", "GyroDevRef"=w178) -> ()  [unwired: 8 in, 2 out]
  n90 = call-poly <vilib>:"WPI_CounterToDigitalSource.vi"("DigitalInputDevRef"=w55) -> ("Digital Source"=w59:T19)  [unwired: 6 out]
  n91 = call-poly <vilib>:"WPI_CounterToDigitalSource.vi"("DigitalInputDevRef"=w56) -> ("Digital Source"=w60:T19)  [unwired: 6 out]
  n92 = call <vilib>:"WPI_CompressorOpen.vi"() -> ("CompressorDevRef"=w1:T28)  [unwired: 14 in, 1 out]
  n93 = call <vilib>:"WPI_EncoderOpen.vi"("DistancePerCount"=0.000488, "Decoding Type"=WPI_EncoderType."2x", "BSource"=w60, "ASource"=w59) -> ("EncoderDevRef"=w54:T23)  [unwired: 6 in, 1 out]
  n94 = call <vilib>:"WPI_EncoderRefNum Registry Set.vi"("refnum name"="Shooter", "EncoderDevRef"=w54) -> ()  [unwired: 8 in, 2 out]
  n95 = call <vilib>:"WPI_CompressorRefNum Registry Set.vi"("refnum name"="Compressor", "CompressorDevRef"=w1) -> ()  [unwired: 8 in, 2 out]
  n96 = call <vilib>:"WPI_DriverStationGet Alliance Info.vi"() -> ("Alliance"=w44:T3)  [unwired: 6 in, 5 out]
  n97 = call <vilib>:"Color Sensor V3 Open.vi"("I2C Bus"=i2c_bus."I2C On-Board") -> ("error out"=w37:errorcluster, "ColorSensorDevRef"=w35:T29)  [unwired: 9 in]
  n98 = call <vilib>:"Color Sensor V3 RefNum Registry Set.vi"("error in (no error)"=w37, "refnum name"="ColorBall", "ColorSensorDevRef"=w35) -> ()  [unwired: 7 in, 2 out]
  n99 = call-poly <vilib>:"WPI_SwitchOpen.vi"("DIO Channel"=FPGA_DIOChannel."DIO 4") -> ("SwitchDevRef"=w25:T31)  [unwired: 9 in, 1 out]
  n100 = call-poly <vilib>:"WPI_SolenoidOpen.vi"("Reverse Solenoid Channel"=WPI_SolenoidChannel."Solenoid 0", "Forward Solenoid Channel"=WPI_SolenoidChannel."Solenoid 1") -> ("SolenoidDevRef"=w114:T32)  [unwired: 8 in, 1 out]
  n101 = call-poly <vilib>:"WPI_SolenoidOpen.vi"("Reverse Solenoid Channel"=WPI_SolenoidChannel."Solenoid 6", "Forward Solenoid Channel"=WPI_SolenoidChannel."Solenoid 7") -> ("SolenoidDevRef"=w110:T32)  [unwired: 8 in, 1 out]
  n102 = Equal?(x=w44, y=WPI_DriverStationAllianceInfo."Red") -> (x = y?=w41:bool)
  n103 = Equal?(x=w44, y=WPI_DriverStationAllianceInfo."Blue") -> (x = y?=w40:bool)
  n104 = call <vilib>:"WPI_SolenoidRefNum Registry Set.vi"("refnum name"="Intake", "SolenoidDevRef"=w114) -> ()  [unwired: 8 in, 2 out]
  n105 = call <vilib>:"WPI_SolenoidRefNum Registry Set.vi"("refnum name"="Climber", "SolenoidDevRef"=w110) -> ()  [unwired: 8 in, 2 out]
  n106 = case shown="True" w41 {
    tunnel: [w218 "Red"] -> w39
    tunnel: [w217 "Blue"] -> w38
    tunnel: w40 -> [w219 _]
    frame False {
      n107 = case shown="False" w219 {
        tunnel: [w220 "Blue"] -> w218
        tunnel: [w220 "Red"] -> w217
        frame False {
          w220 = "No Data"
        }
        frame True {
        }
      }
    }
    frame True {
    }
  }
  n108 = call <vilib>:"WPI_SwitchRefNum Registry Set.vi"("refnum name"="IRConveyor", "SwitchDevRef"=w25) -> ()  [unwired: 8 in, 2 out]
  n109 = call <vilib>:"Color Sensor V3 Add Color Match.vi"("Color"="Blue Calibration", "Name"="Blue") -> ()  [unwired: 10 in]
  n110 = call <vilib>:"Color Sensor V3 Add Color Match.vi"("Color"="Red Calibration", "Name"="Red") -> ()  [unwired: 10 in]
  n111 = global write "StateMachineOperation.vi" "Ball Color"(w39) -> ()
  n112 = global write "StateMachineOperation.vi" "Opposite Color"(w38) -> ()
  n113 = call-poly <vilib>:"WPI_SwitchOpen.vi"("DIO Channel"=FPGA_DIOChannel."DIO 7") -> ("SwitchDevRef"=w20:T31)  [unwired: 9 in, 1 out]
  n114 = call <vilib>:"Color Sensor V3 Add Color Match.vi"("Color"="Nothing", "Name"="Nothing") -> ()  [unwired: 10 in]
  n115 = call <vilib>:"WPI_SwitchRefNum Registry Set.vi"("refnum name"="SwitchHood", "SwitchDevRef"=w20) -> ()  [unwired: 8 in, 2 out]
  "error out" <- "error in"
